vi "Test Smoothing.vi"() -> ()   [LabVIEW 2013]
panel:
  out "Waveform Chart":dbl(graph)
  in  "Slide":dbl(slide) scale=0.0..100.0
  in  "Warming up?":bool
  in  "Number to Average":i32=30
  in  "Boolean":bool
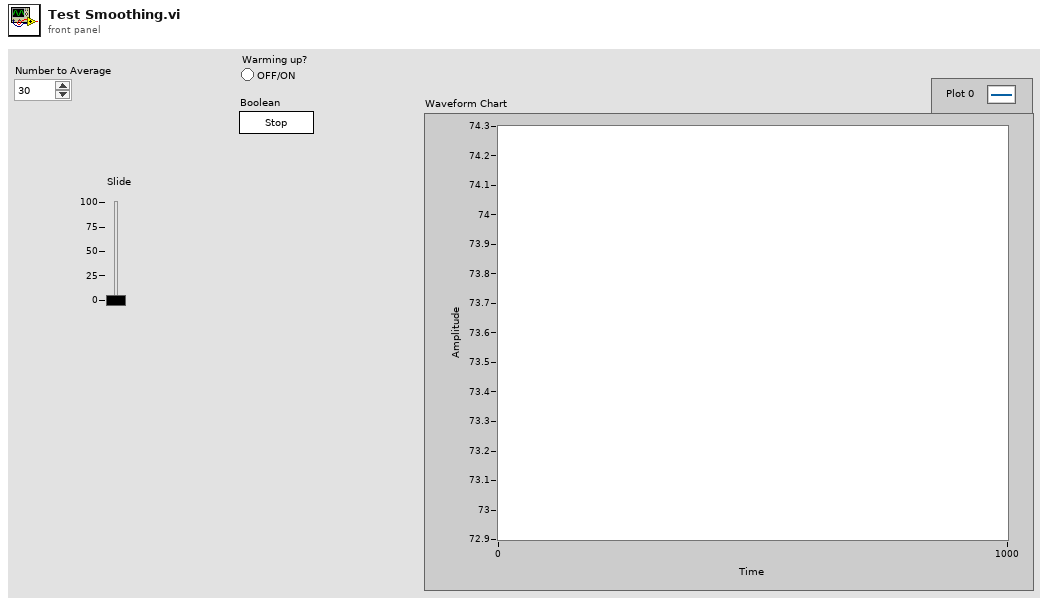
[diagram p1: front panel]
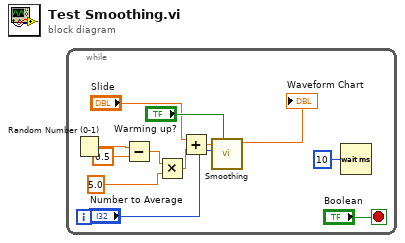
[diagram p0: block diagram]
diagram:
  n1 = while {
    stop <- "Boolean" stop-if-true
    n2 = Random Number (0-1)() -> (number: 0 to 1=w9:dbl)
    n3 = Subtract(x=w9, y=0.5) -> (x-y=w7:dbl)
    n4 = Multiply(x=w7, y=5.0) -> (x*y=w5:dbl)
    n5 = Add(x="Slide", y=w5) -> (x+y=w3:dbl)
    n6 = call "Smoothing.vi"("Warming up?"="Warming up?", "Number to Average"="Number to Average", "O2%"=w3) -> ("Mean O2%"=→"Waveform Chart":dbl)  [unwired: 8 in]
    n7 = Wait (ms)(milliseconds to wait=u32 10) -> ()  [unwired: 1 out]
  }
